vi "Dispense_mirrored.vi"(8 "error in (no error)":errorcluster, 10 "Bottom Pin":tag="A/PWM1", 11 "Top Pin":tag="A/PWM0") -> (0 "error out":errorcluster, 3 "Finished":bool)   [LabVIEW 2014]
uses:
  Controls/Dispenser Functions.ctl
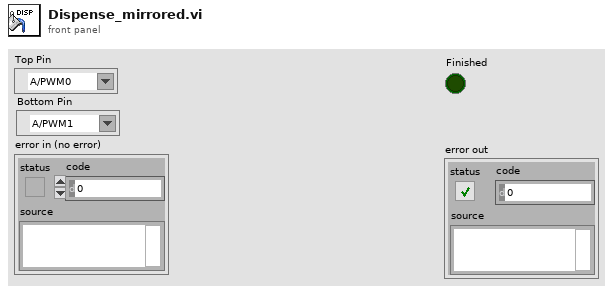
[diagram p1: front panel]
types:
  T1 = typedef "Dispenser Functions.ctl" = enum16{"Open Top", "Close Top", "Close Bottom", "Open Bottom"}
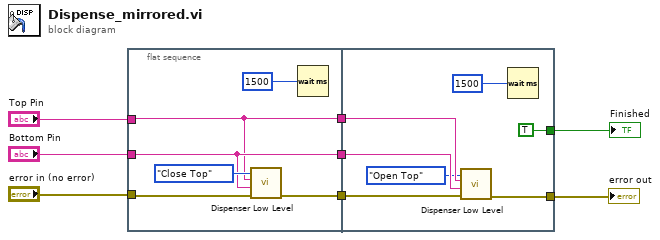
[diagram p0: block diagram]
diagram:
  n1 = flat-sequence {
    tunnel: [w10] -> w8
    tunnel: [w9] -> w7
    tunnel: [w12] -> w6
    tunnel: "error in (no error)" -> [w11]
    tunnel: "Bottom Pin" -> [w10]
    tunnel: "Top Pin" -> [w9]
    tunnel: w8 -> [w17]
    tunnel: w7 -> [w18]
    tunnel: w6 -> [w20]
    tunnel: [w19] -> w5
    tunnel: [TRUE ("Finished")] -> w4
    frame #0 {
      n2 = call "Dispenser Low Level.vi"("error in (no error)"=w11, "Bottom Pin"=w10, "Top Pin"=w9, "Function"=Dispenser_Functions."Close Top") -> ("error out"=w12:errorcluster)  [unwired: 7 in]
      n3 = Wait (ms)(milliseconds to wait=u32 1500) -> ()  [unwired: 1 out]
    }
    frame #1 {
      n4 = call "Dispenser Low Level.vi"("error in (no error)"=w20, "Bottom Pin"=w17, "Top Pin"=w18, "Function"=Dispenser_Functions."Open Top") -> ("error out"=w19:errorcluster)  [unwired: 7 in]
      n5 = Wait (ms)(milliseconds to wait=u32 1500) -> ()  [unwired: 1 out]
    }
  }
  "error out" <- w5
  "Finished" <- w4
